vi "SD_selector.vi"(7 "myGateCC":dbl, 8 "myDrainCC":dbl, 9 "myVvar":dbl, 10 "SMU_1_port":string) -> (0 "myCC2":dbl, 1 "myCC1":dbl, 2 "myV2":dbl, 3 "myV1":dbl)   [LabVIEW 2021]
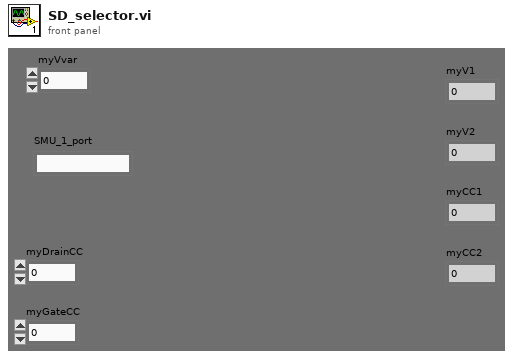
[diagram p1: front panel]
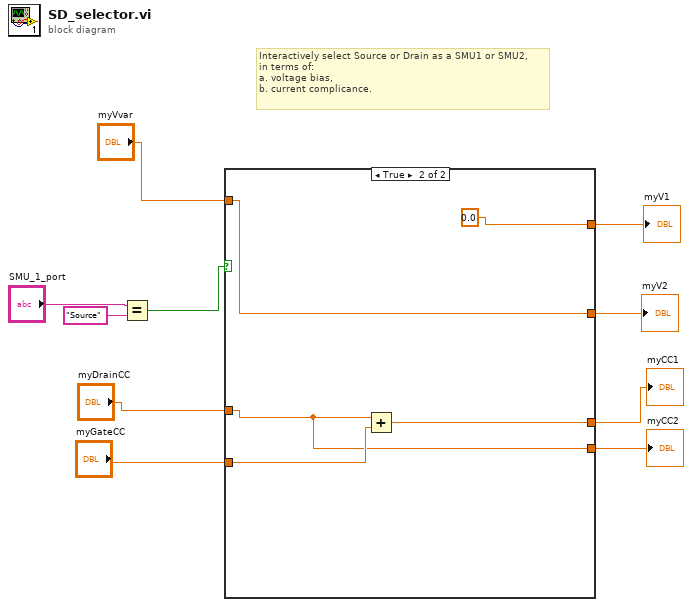
[diagram p0: block diagram]
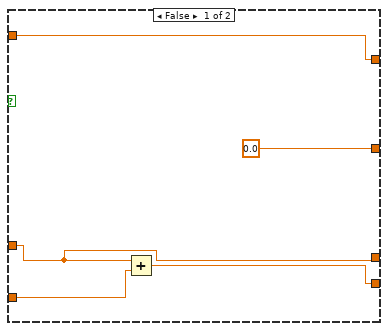
[diagram p2: hidden frame]
diagram:
  # "Interactively select Source or Drain as a SMU1 or SMU2,\nin terms of:\na. voltage bias,\nb. current complicance."
  n1 = Equal?(x="SMU_1_port", y="Source") -> (x = y?=w8:bool)
  n2 = case shown="True" w8 {
    tunnel: [w14 0.0] -> w7
    tunnel: [0.0 w19] -> w6
    tunnel: "myVvar" -> [w14 w19]
    tunnel: "myDrainCC" -> [w11 w16]
    tunnel: "myGateCC" -> [w13 w18]
    tunnel: [w11 w17] -> w2
    tunnel: [w12 w16] -> w1
    frame False {
      n3 = Add(x=w11, y=w13) -> (x+y=w12:dbl)
    }
    frame True {
      n4 = Add(x=w16, y=w18) -> (x+y=w17:dbl)
    }
  }
  "myV1" <- w7
  "myV2" <- w6
  "myCC1" <- w2
  "myCC2" <- w1
